vi "test Parameter Initialization.vi"(8 "error in (no error)":errorcluster, 11 "TestCase in":refnum<class "Switch Consumer Test Case.lvclass">) -> (0 "error out":errorcluster, 3 "TestCase out":refnum<class "Switch Consumer Test Case.lvclass">)   [LabVIEW 2017, in "Switch Consumer Test Case.lvclass"]
uses:
  Switch Consumer Test Case.lvclass
  Support/Switch/Test Switch Consumer/Test Switch Consumer.lvclass
  Switch Consumer Test Case.lvclass/Switch Consumer Test Case.ctl
  Support/Switch/Test Switch Consumer/Test Switch Consumer.lvclass/Test Switch Consumer.ctl
  Support/Switch/Test Switch Consumer/Read Test Param.vi
  <vilib>/addons/_JKI Toolkits/VI Tester/TestCase.llb/TestCase.lvclass
  C:/Program Files (x86)/National Instruments/LabVIEW 2017/vi.lib/addons/_JKI Toolkits/VI Tester/TestCase.llb/TestCase.lvclass
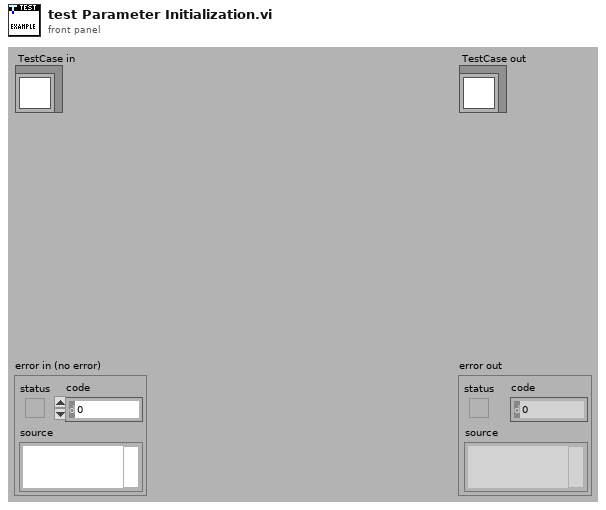
[diagram p1: front panel]
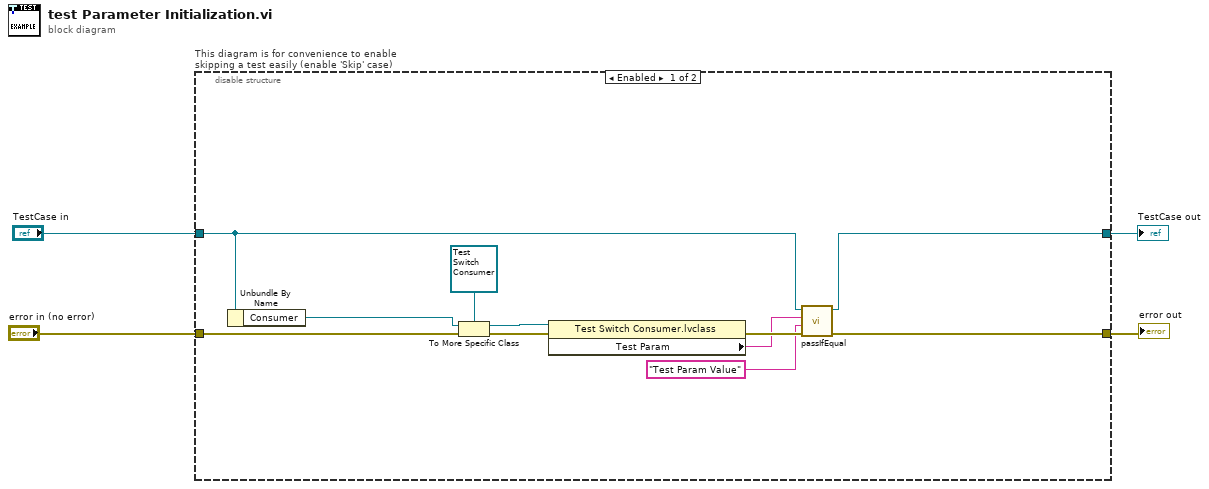
[diagram p0: block diagram]
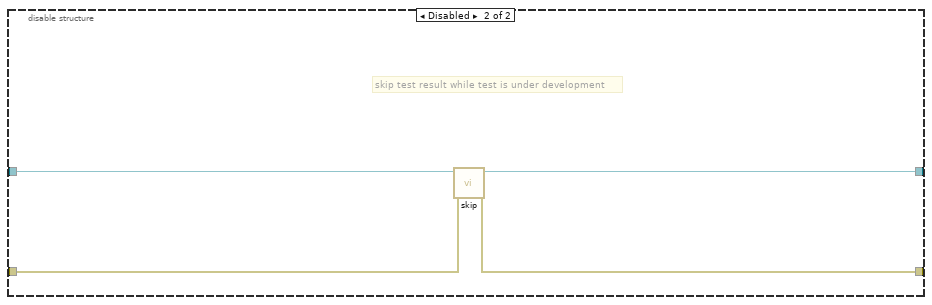
[diagram p2: hidden frame]
diagram:
  n1 = disable-structure "This diagram is for convenience to enable skipping a test easily (enable 'Skip' case)" shown="Enabled" {
    disable-tunnel: "TestCase in" -> [w6 w19]
    disable-tunnel: [w5 w17] -> w1
    disable-tunnel: [w9 w18] -> w3
    disable-tunnel: "error in (no error)" -> [w15 w16]
    frame Enabled {
      n2 = Unbundle By Name(w6) -> ("Consumer"=w14:refnum<class "Abstract Consumer.lvclass">)
      n3 = To More Specific Class(target class=refnum<class "Test Switch Consumer.lvclass"> refnum ("Test Switch Consumer.lvclass"), reference=w14, error in=w15) -> (specific class reference=w12:refnum<class "Test Switch Consumer.lvclass">, error out=w11:errorcluster)
      n4 = property class="Test Switch Consumer.lvclass"(reference=w12, error in=w11) -> (error out=w10:errorcluster, "Test Param"=w8:string)  [unwired: 1 out]
      n5 = call-dynamic "passIfEqual.vi"("error in (no error)"=w10, "y"="Test Param Value" ("Topology"), "x"=w8, "TestCase in"=w6) -> ("error out"=w9:errorcluster, "TestCase out"=w5:refnum<class "Switch Consumer Test Case.lvclass">)  [unwired: 6 in]
    }
    frame Disabled {
      # "skip test result while test is under development"
      n6 = call <vilib>:"skip.vi"("error in (no error)"=w16, "TestCase in"=w19) -> ("error out"=w18:errorcluster, "TestCase out"=w17:refnum<class "Switch Consumer Test Case.lvclass">)  [unwired: 8 in]
    }
  }
  "error out" <- w3
  "TestCase out" <- w1
